vi "Ramp.vi"(8 "Force?":bool, 9 "Force":dbl, 10 "Rate":dbl, 11 "Target":dbl) -> (2 "Output":dbl)   [LabVIEW 2014]
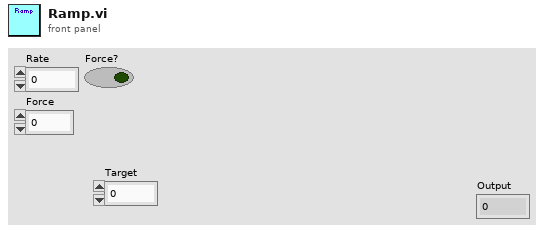
[diagram p1: front panel]
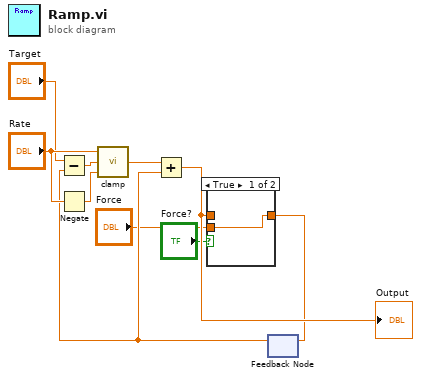
[diagram p0: block diagram]
diagram:
  n1 = Negate(x="Rate") -> (-x=w10:dbl)
  n2 = feedback #1() -> (w5:dbl)  [unwired: 1 in]
  n3 = Subtract(x="Target", y=w5) -> (x-y=w7:dbl)
  n4 = call "clamp.vi"("Min"=w10, "Input"=w7, "Max"="Rate") -> ("Output"=w6:dbl)
  n5 = Add(x=w6, y=w5) -> (x+y=w4:dbl)
  "Output" <- w4
  n6 = case shown="True" "Force?" {
    tunnel: [w11 w12] -> w3
    tunnel: w4 -> [_ w12]
    tunnel: "Force" -> [w11 _]
    frame True {
    }
    frame False {
    }
  }
  n7 = feedback-in #1(w3) -> ()
